vi "database_connection_write_EVO.vi"(5 "ODBC data source name":string="amrc_monitoring", 6 "error in (no error)":errorcluster, 7 "G1?":u32, 8 "current time":timestamp, 9 "data 2":dbl[](array[numeric]), 10 "Machine Data":T1={"Zload"="", "Yload"="", "Xload"="", "path_position"="", "Fovr"="", "SspeedOvr"="", "Program Name"="", "Program status"="", "Block of code being executed"="", "Line of code"="", "Machine availability"="", "Emergency status"="", "Controller mode"="", "Tool_id"="UNAVAILABLE"}, 11 "Machine type":string) -> (3 "error out":errorcluster)   [LabVIEW 2017]
uses:
  <vilib>/addons/database/Connection.llb/DB Tools Open Connec (Path).vi
  <vilib>/addons/database/Connection.llb/Conn Execute.vi
  <vilib>/addons/database/Recordset.llb/Rec Destroy - Connection.vi
  <vilib>/regexp/Match Regular Expression.xnode
  <vilib>/addons/database/NI_Database_API.lvlib
panel:
  out "string":string="(timestamp,machine_status,g1,tool_id,force_acc_raw_data,spike_raw_data,spindle_load,spindle_speed,feed_rate,I,J,K,X,Y,Z,position_A,position_B ,Xload,Yload,Zload,Aload,Bload,program_number,accel_x_rms,accel_y_rms,accel_z_rms,force_x_rms,force_y_rms,force_z_rms,axial_force_rms, torque_rms,bending_x_rms,bending_y_rms,estop,block_code,fovr,sspeedovr,program_name,line) VALUES ("
  out "data 3":dbl[](array[numeric])
  out "path_position":string
  out "x = y?":bool
  out "submatch 1":string
  out "after match 3":string
  out "empty? 2":bool
  out "after match 2":string
  out "resulting string 4":string
  out "Xload":string
  out "concatenated string 6":string
  out "resulting string 3":string
  out "concatenated string 2":string
  out "resulting string 2":string
  out "ODBC data source name 2":string="amrc_monitoring"
  out "resulting string":string
  out "size(s)":i32
  out "concatenated string 5":string
  out "concatenated string 3":string
  out "concatenated string":string
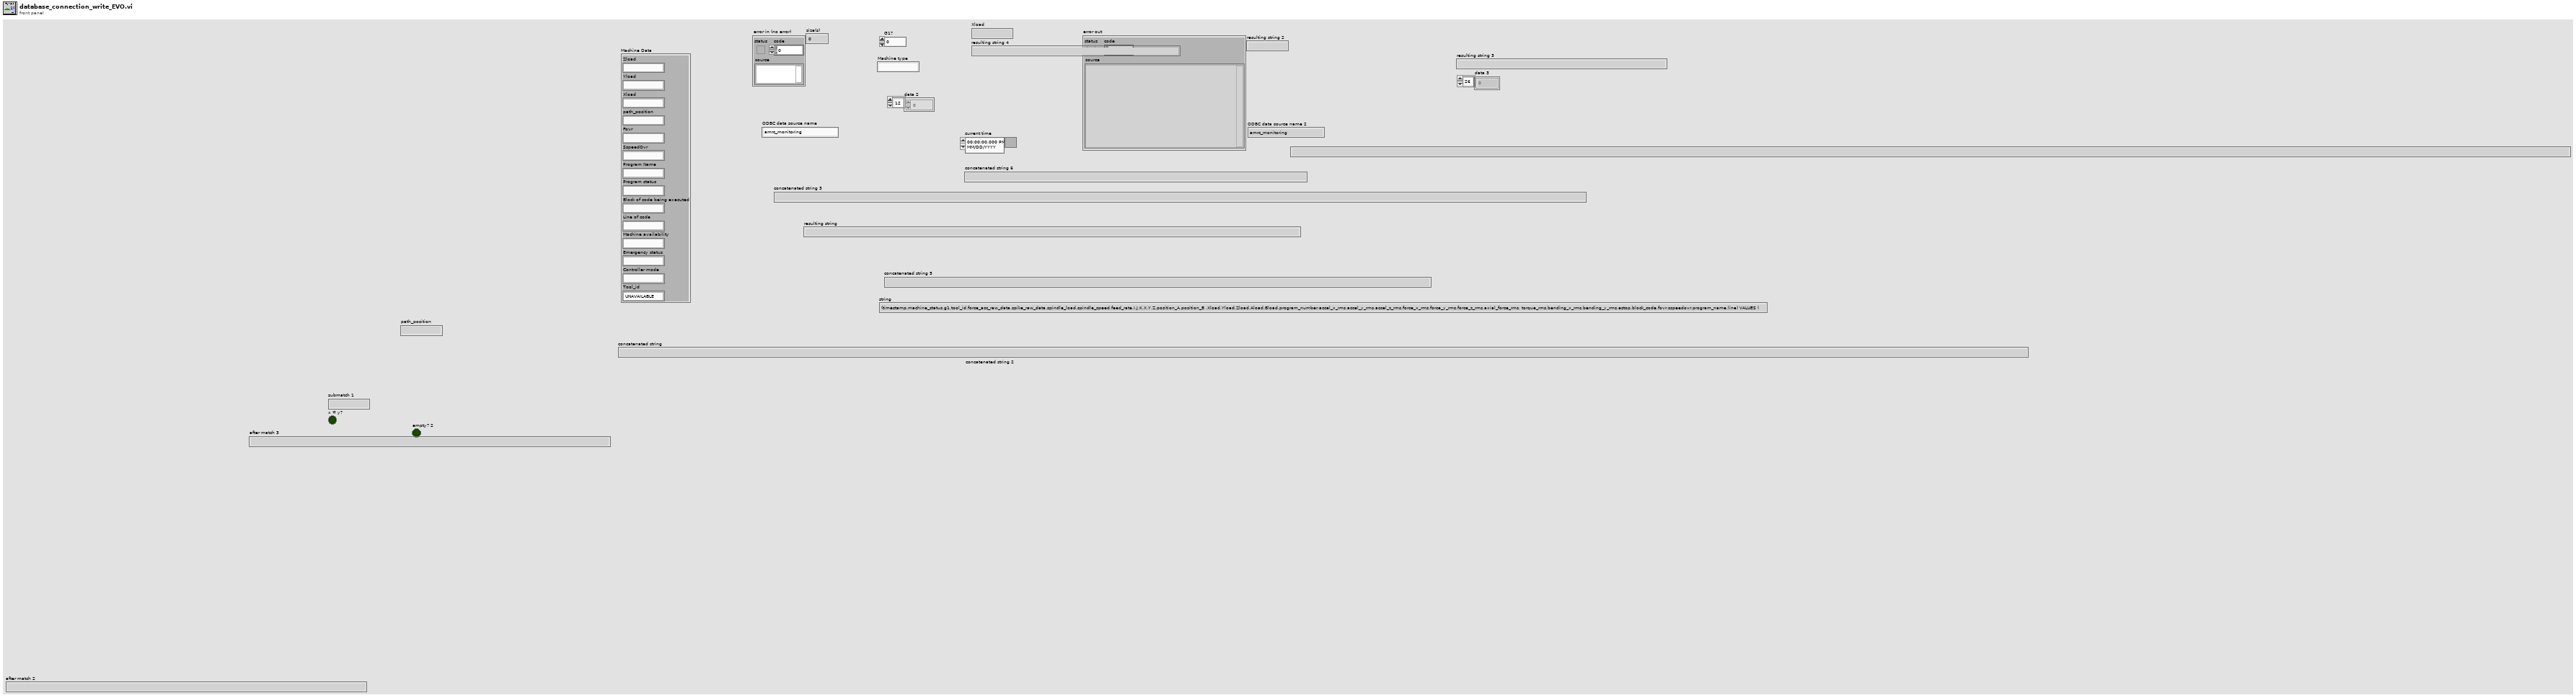
[diagram p1: front panel]
types:
  T1 = cluster{"Zload":string, "Yload":string, "Xload":string, "path_position":string, "Fovr":string, "SspeedOvr":string, "Program Name":string, "Program status":string, "Block of code being executed":string, "Line of code":string, "Machine availability":string, "Emergency status":string, "Controller mode":string, "Tool_id":string}
  T2 = typedef "NI_Database_API.lvlib/Conn ObjectReference.ctl" = refnum<k1>
  T3 = typedef "NI_Database_API.lvlib/Rec ObjectReference.ctl" = refnum<k1>
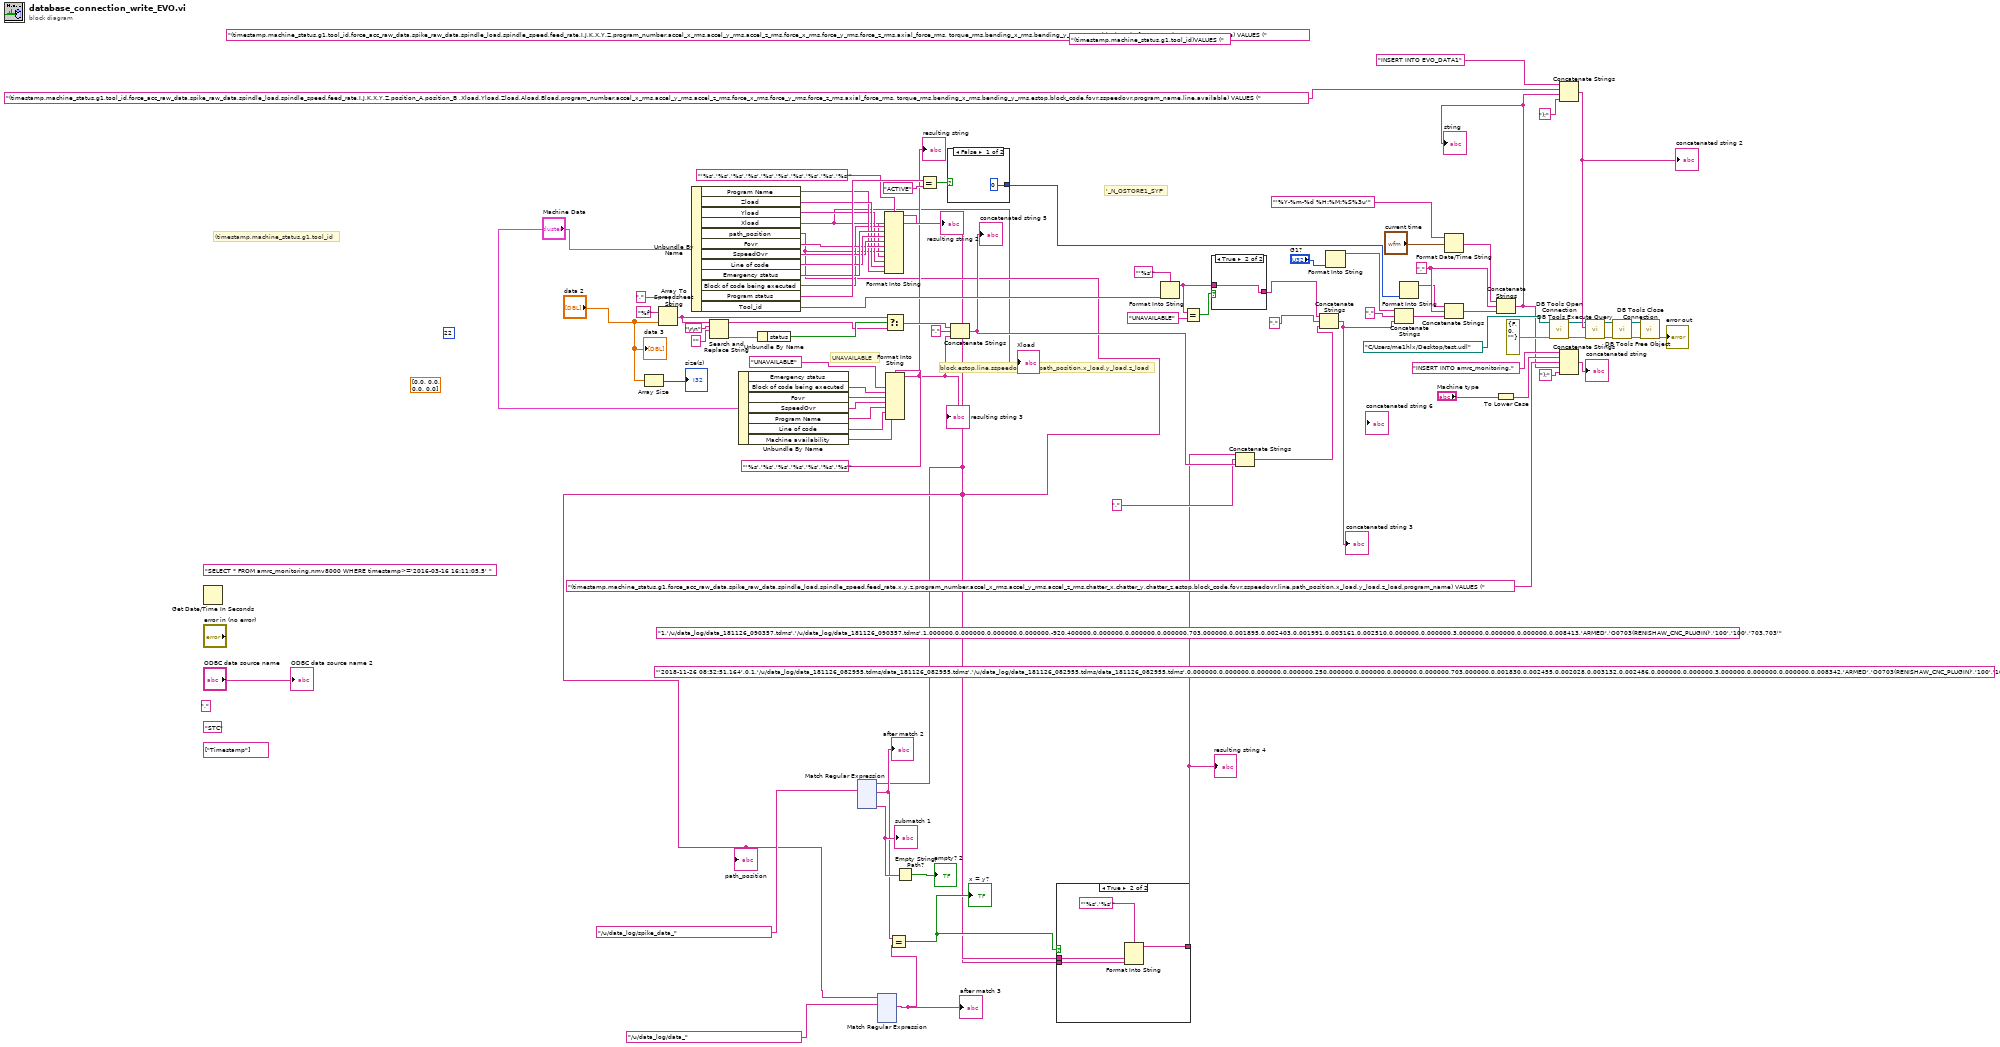
[diagram p0: block diagram]
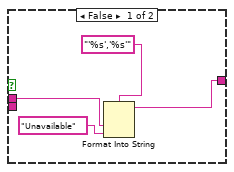
[diagram p2: hidden frame]
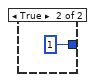
[diagram p4: hidden frame]
diagram:
  (unwired) "(timestamp,machine_status,g1,tool_id,force_acc_raw_data,spike_raw_data,spindle_load,spindle_speed,feed_rate,I,J,K,X,Y,Z,program_number,accel_x_rms,accel_y_rms,accel_z_rms,force_x_rms,force_y_rms,force_z_rms,axial_force_rms, torque_rms,bending_x_rms,bending_y_rms,estop,block_code,fovr,sspeedovr,program_name) VALUES (" ("string")
  (unwired) "(timestamp,machine_status,g1,tool_id)VALUES (" ("string")
  (unwired) dbl[] [0.0, 0.0, 0.0, 0.0]
  (unwired) "1,'/u/data_log/data_181126_090357.tdms','/u/data_log/data_181126_090357.tdms',1.000000,0.000000,0.000000,0.000000,-920.400000,0.000000,0.000000,0.000000,703.000000,0.001895,0.002403,0.001991,0.003161,0.002510,0.000000,0.000000,3.000000,0.000000,0.000000,0.008413,'ARMED','O0703(RENISHAW_CNC_PLUGIN)','100','100','703.703'" ("concatenated string 4")
  (unwired) "'2018-11-26 08:32:51.164',0,1,'/u/data_log/data_181126_082955.tdms/data_181126_082955.tdms','/u/data_log/data_181126_082955.tdms/data_181126_082955.tdms',0.000000,0.000000,0.000000,0.000000,250.000000,0.000000,0.000000,0.000000,703.000000,0.001830,0.002455,0.002028,0.003132,0.002486,0.000000,0.000000,3.000000,0.000000,0.000000,0.008342,'ARMED','O0703(RENISHAW_CNC_PLUGIN)','100','100','703.703'" ("concatenated string 2")
  (unwired) 22
  (unwired) "," ("string")
  (unwired) string[] ["Timestamp"]
  (unwired) "STC"
  w47 = "," ("string")
  (unwired) "SELECT * FROM amrc_monitoring.nmv8000 WHERE timestamp>='2016-03-16 16:11:05.5' " ("SQL query")
  # "(timestamp,machine_status,g1,tool_id"
  # "'_N_OSTORE1_SYF'"
  # "UNAVAILABLE"
  # "block,estop,line,sspeedovr,fovr,path_position,x_load,y_load,z_load"
  n1 = Get Date/Time In Seconds() -> ()  [unwired: 1 out]
  n2 = Array Size(array="data 2") -> (size(s)=→"size(s)":i32)
  n3 = Array To Spreadsheet String(delimiter (Tab)=",", array="data 2", 3:"%f" ("format string")) -> (spreadsheet string=w73:string)
  n4 = Unbundle By Name("Machine Data") -> ("Program Name"=w60:string, "Zload"=w64:string, "Yload"=w25:string, "Xload"=w6:string, "path_position"=w7:string, "Fovr"=w65:string, "SspeedOvr"=w66:string, "Line of code"=w67:string, "Emergency status"=w68:string, "Block of code being executed"=w58:string, "Program status"=w86:string, "Tool_id"=w52:string)
  "Xload" <- w6
  "path_position" <- w7
  n5 = Search and Replace String(input string=w73, search string="\r\n", replace string="" ("replace string (\"\")")) -> (result string=w74:string, error out=w76:errorcluster)  [unwired: 5 in, 2 out]
  n6 = Unbundle By Name("Machine Data") -> ("Block of code being executed"=w32:string, "Fovr"=w31:string, "SspeedOvr"=w30:string, "Program Name"=w29:string, "Line of code"=w4:string, "Machine availability"=w1:string)  [unwired: 1 out]
  n7 = Unbundle By Name(w76) -> ("status"=w75:bool)
  n8 = xnode "Match Regular Expression"("input string"=w6, "regular expression"="/u/data_log/spike_data_") -> ("after match"=w10:string, "submatch 1"=w11:string)  [unwired: 4 in, 4 out]
  "after match 2" <- w10
  "submatch 1" <- w11
  n9 = xnode "Match Regular Expression"("input string"=w7, "regular expression"="/u/data_log/data_") -> ("after match"=w9:string)  [unwired: 4 in, 5 out]
  "after match 3" <- w9
  n10 = Format Into String(format string="'%s','%s','%s','%s','%s','%s','%s','%s','%s','%s'", w58, w68, w67, w66, w65, w7, w6, w25, w64, w60) -> (resulting string=→"resulting string 2":string)  [unwired: 2 in, 1 out]
  n11 = Select(t=w73, s=w75, f=w74) -> (s? t:f=w61:string)
  n12 = Format Into String(format string="'%s','%s','%s','%s','%s','%s','%s'", "UNAVAILABLE" ("format string"), w32, w31, w30, w29, w4, w1) -> (resulting string=w24:string)  [unwired: 2 in, 1 out]
  "resulting string" <- w24
  "resulting string 3" <- w24
  n13 = Equal?(x=w10, y=w9) -> (x = y?=w8:bool)
  "x = y?" <- w8
  n14 = Empty String/Path?(string/path=w11) -> (empty?=→"empty? 2":bool)
  n15 = Equal?(x=w86, y="ACTIVE") -> (x = y?=w84:bool)
  n16 = case shown="False" w84 {
    tunnel: [0 1] -> w21
    frame False {
    }
    frame True {
    }
  }
  n17 = Concatenate Strings(w61, "," ("string"), w24) -> (w18:string)
  "concatenated string 5" <- w18
  n18 = case shown="True" w8 {
    tunnel: w7 -> [w93 w95]
    tunnel: w6 -> [_ w98]
    tunnel: [w92 w96] -> w5
    frame False {
      n19 = Format Into String(format string="'%s','%s'", w93, "Unavailable" ("Tool_id")) -> (resulting string=w92:string)  [unwired: 2 in, 1 out]
    }
    frame True {
      n20 = Format Into String(format string="'%s','%s'", w95, w98) -> (resulting string=w96:string)  [unwired: 2 in, 1 out]
    }
  }
  "resulting string 4" <- w5
  n21 = Format Into String(format string="'%s'", w52) -> (resulting string=w51:string)  [unwired: 2 in, 1 out]
  n22 = Equal?(x=w51, y="UNAVAILABLE") -> (x = y?=w83:bool)
  n23 = case shown="True" w83 {
    tunnel: w51 -> [w99 w100]
    tunnel: [w99 w100] -> w2
    frame False {
    }
    frame True {
    }
  }
  n24 = Concatenate Strings(w5, "," ("string"), w18) -> (w16:string)
  n25 = Concatenate Strings(w2, "," ("string"), w16) -> (w22:string)
  "concatenated string 3" <- w22
  n26 = Format Into String("G1?") -> (resulting string=w45:string)  [unwired: 3 in, 1 out]
  n27 = Concatenate Strings(w45, "," ("string"), w22) -> (w23:string)
  n28 = Format Into String(w21) -> (resulting string=w46:string)  [unwired: 3 in, 1 out]
  n29 = Concatenate Strings(w46, w47, w23) -> (w79:string)
  n30 = Format Date/Time String(time format string (%c)="'%Y-%m-%d %H:%M:%S%3u'", seconds (now)="current time") -> (date/time string=w48:string)  [unwired: 1 in]
  n31 = To Lower Case(string="Machine type") -> (all lower case string=w70:string)
  n32 = Concatenate Strings(w48, w47, w79) -> (w3:string)
  "string" <- w3
  n33 = call-poly <vilib>:"DB Tools Open Connection.vi"("error in (no error)"=errorcluster {"status"=FALSE, "code"=0, "source"=""}, "connection information"=path "C:/Users/me1hlx/Desktop/test.udl") -> ("error out"=w43:errorcluster, "connection reference"=w37:T2)  [unwired: 6 in]
  n34 = Concatenate Strings("INSERT INTO EVO_DATA1" ("string"), "(timestamp,machine_status,g1,tool_id,force_acc_raw_data,spike_raw_data,spindle_load,spindle_speed,feed_rate,I,J,K,X,Y,Z,position_A,position_B ,Xload,Yload,Zload,Aload,Bload,program_number,accel_x_rms,accel_y_rms,accel_z_rms,force_x_rms,force_y_rms,force_z_rms,axial_force_rms, torque_rms,bending_x_rms,bending_y_rms,estop,block_code,fovr,sspeedovr,program_name,line,available) VALUES (" ("string"), w3, ");" ("string")) -> (w44:string)
  "concatenated string 2" <- w44
  n35 = Concatenate Strings("INSERT INTO amrc_monitoring." ("string"), w70, "(timestamp,machine_status,g1,force_acc_raw_data,spike_raw_data,spindle_load,spindle_speed,feed_rate,x,y,z,program_number,accel_x_rms,accel_y_rms,accel_z_rms,chatter_x,chatter_y,chatter_z,estop,block_code,fovr,sspeedovr,line,path_position,x_load,y_load,z_load,program_name) VALUES (" ("string"), w3, ");" ("string")) -> (→"concatenated string":string)
  n36 = call-poly <vilib>:"DB Tools Execute Query.vi"("error in (no error)"=w43, "SQL query"=w44, "connection reference"=w37) -> ("error out"=w40:errorcluster, "recordset reference"=w41:T3)  [unwired: 5 in]
  n37 = call-poly <vilib>:"DB Tools Free Object.vi"("error in (no error)"=w40, "recordset reference"=w41) -> ("error out"=w38:errorcluster, "connection reference"=w39:T2)  [unwired: 8 in]
  n38 = call <vilib>:"DB Tools Close Connection.vi"("error in (no error)"=w38, "connection reference"=w39) -> ("error out"=→"error out":errorcluster)  [unwired: 5 in]
  "ODBC data source name 2" <- "ODBC data source name"
  "data 3" <- "data 2"
